vi "BGAndSrewImage.vi"(8 "error in (no error)":errorcluster, 9 "BG Image":T1, 10 "Image":T1, 11 "S arrays.S 0":i32[][](array[numeric])) -> (0 "error out":errorcluster, 1 "empty image":bool, 3 "Image Out":T1, 4 "time 2":u32)   [LabVIEW 2011]
uses:
  IMAQ Image.ctl
  NI_Vision_Development_Module.lvlib
panel:
  out "time:filter":u32
  out "time:screw":u32
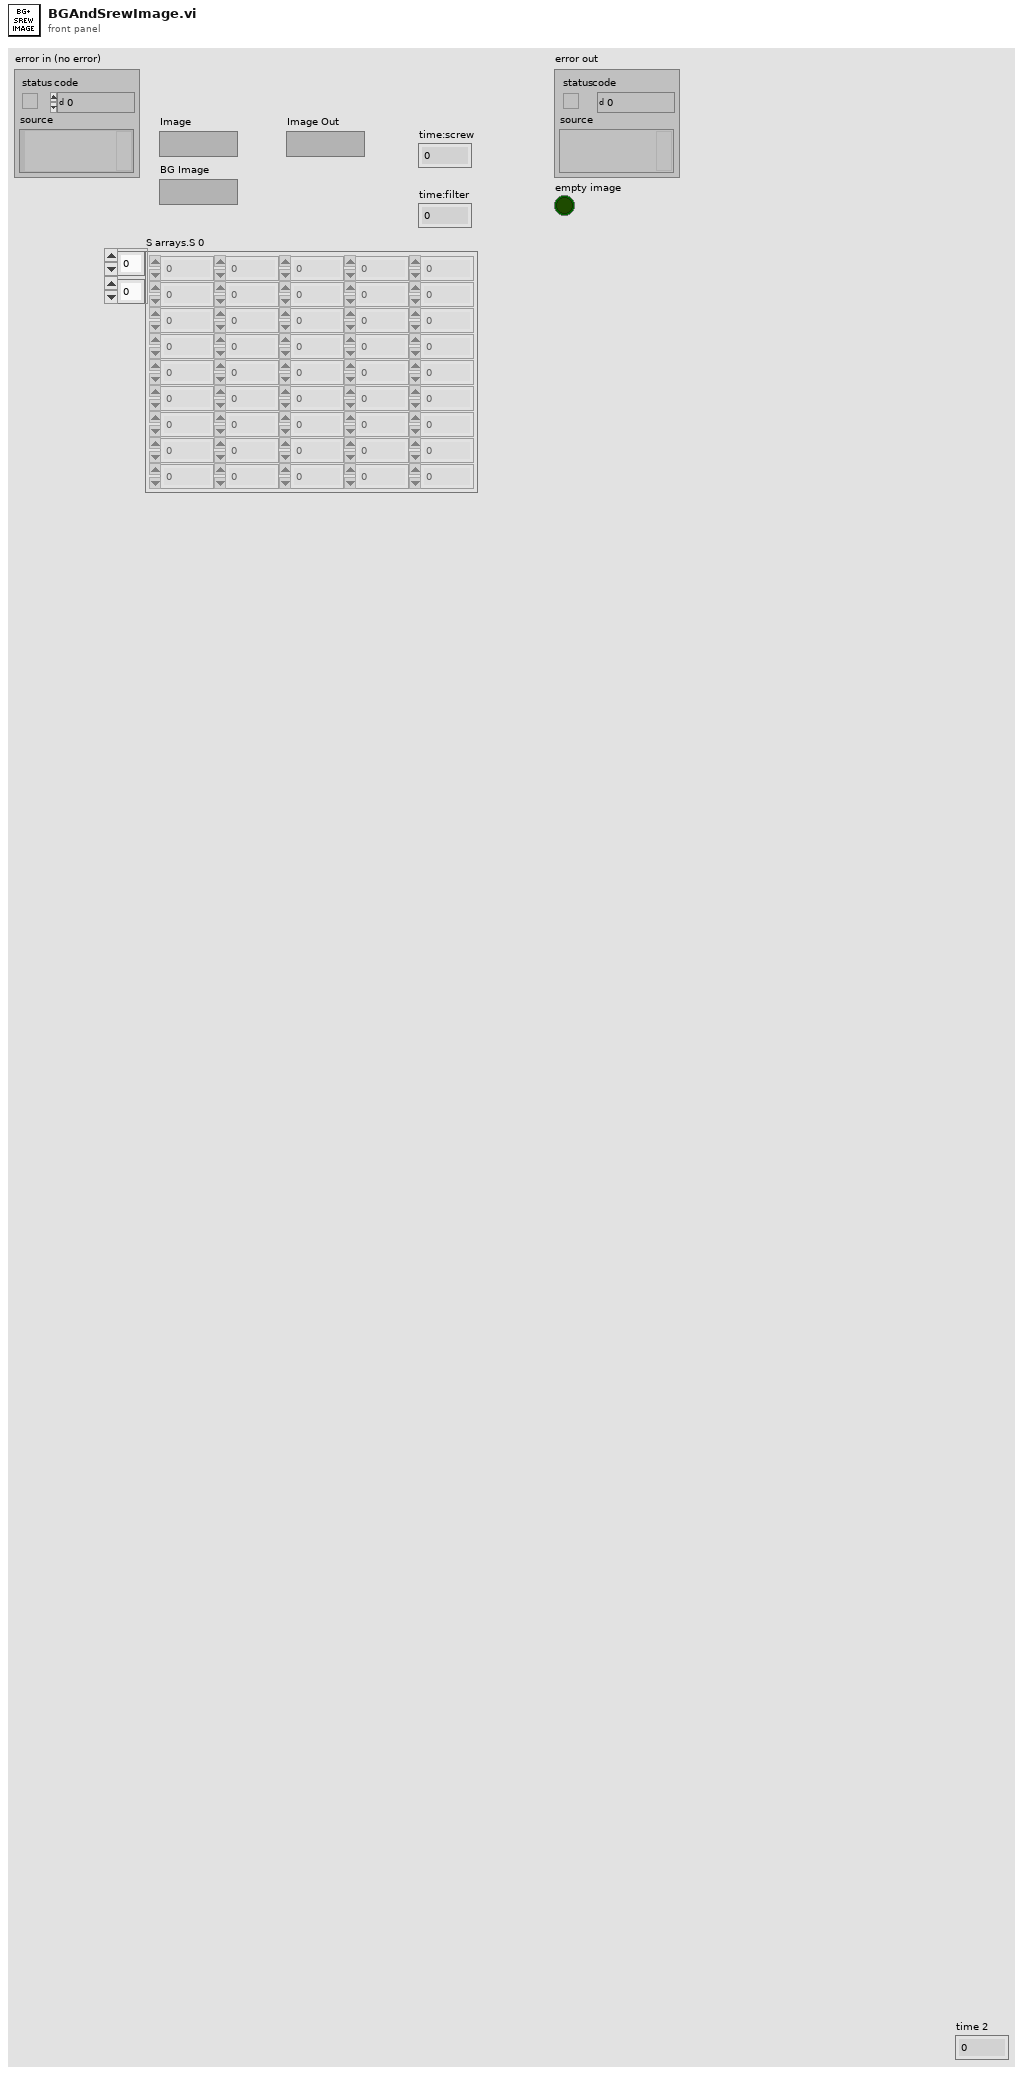
[diagram p1: front panel]
types:
  T1 = typedef "IMAQ Image.ctl" = refnum<image>
  T2 = cluster{"X Size":i32, "Y Size":i32, "Order #":i32}
  T3 = cluster{"X Size":i32, "Y Size":i32, "% Tolerance":i32}
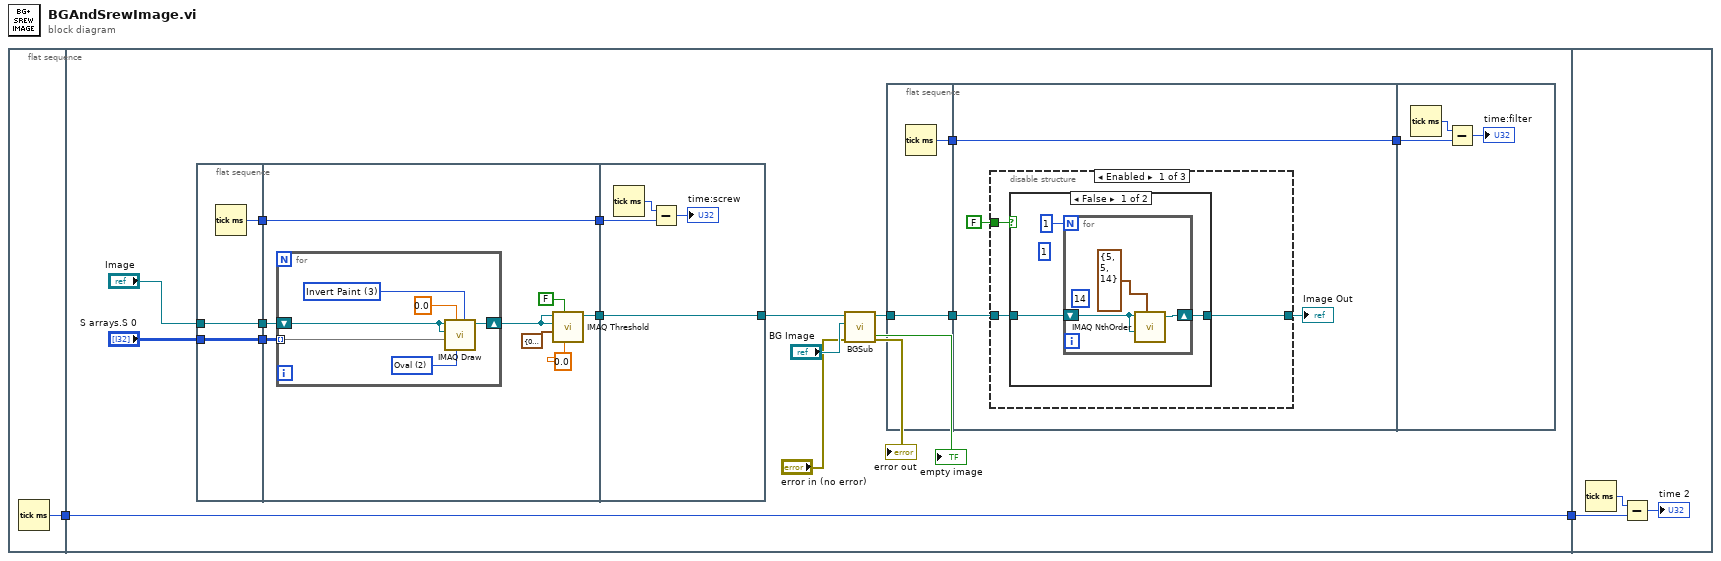
[diagram p0: block diagram]
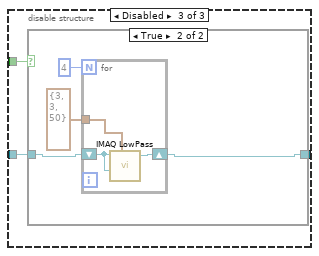
[diagram p4: hidden frame]
diagram:
  n1 = flat-sequence {
    tunnel: [w3] -> w1
    tunnel: [w19] -> w2
    tunnel: w1 -> [w19]
    tunnel: w2 -> [w73]
    frame #0 {
      n2 = Tick Count (ms)() -> (millisecond timer value=w3:u32)
    }
    frame #1 {
      n3 = flat-sequence {
        tunnel: "Image" -> [w53]
        tunnel: "S arrays.S 0" -> [w54]
        tunnel: [w54] -> w17
        tunnel: [w53] -> w16
        tunnel: [w52] -> w15
        tunnel: [w56] -> w18
        tunnel: w17 -> [w62]
        tunnel: w16 -> [w61]
        tunnel: w15 -> [w55]
        tunnel: [w55] -> w14
        tunnel: [w72] -> w10
        tunnel: w18 -> [w72]
        tunnel: w14 -> [w69]
        frame #0 {
          n4 = Tick Count (ms)() -> (millisecond timer value=w52:u32)
        }
        frame #1 {
          n5 = for {
            shift-right: [w67] -> w57
            shift-left: w61 -> [w68]
            tunnel: w62 -> [w64] mode=indexing
            w66 = u16 2 items=["Line", "Rectangle", "Oval"] ("Shape to draw")
            w65 = u16 3 items=["Frame", "Paint", "Invert Frame", "Invert Paint"] ("Draw Mode")
            n6 = call "IMAQ Draw"("Draw Mode"=w65, "Shape to draw"=w66, "Pixel Color"=sgl 0.0, "Coordinates"=w64, "Image Dst"=w68, "Image Src"=w68) -> ("Image Dst Out"=w67:T1)  [unwired: 4 in, 1 out]
          }
          n7 = call "IMAQ Threshold"("Replace Value"=sgl 0.0, "Keep/Replace Value (Replace)"=FALSE, "Range"=cluster{"Lower value":sgl, "Upper value":sgl} {"Lower value"=0.0, "Upper value"=999999.0}, "Image Dst"=w57, "Image Src"=w57) -> ("Image Dst Out"=w56:T1)  [unwired: 5 in, 1 out]
        }
        frame #2 {
          n8 = Tick Count (ms)() -> (millisecond timer value=w70:u32)
          n9 = Subtract(x=w70, y=w69) -> (x-y=→"time:screw":u32)
        }
      }
      n10 = call "BGSub.vi"("error in (no error)"="error in (no error)", "BG IN"="BG Image", "raw Image In"=w10) -> ("error out"=→"error out":errorcluster, "Refnum out"=w9:T1, "empty image"=→"empty image":bool)  [unwired: 6 in]
      n11 = flat-sequence {
        tunnel: w9 -> [w22]
        tunnel: [w22] -> w13
        tunnel: [w21] -> w11
        tunnel: w13 -> [w24]
        tunnel: [w26] -> w12
        tunnel: w11 -> [w26]
        tunnel: w12 -> [w49]
        frame #0 {
          n12 = Tick Count (ms)() -> (millisecond timer value=w21:u32)
        }
        frame #1 {
          n13 = disable-structure shown="Enabled" {
            disable-tunnel: [w28 w37 w39] -> w25
            disable-tunnel: w24 -> [w29 w37 w40]
            disable-tunnel: FALSE ("empty array") -> [w27 _ w38]
            frame Enabled {
              n14 = case shown="False" w27 {
                tunnel: w29 -> [w32 w36]
                tunnel: [w31 w36] -> w28
                frame False {
                  (unwired) 1
                  n15 = for {
                    N: 1 -> [_]
                    shift-right: [w33] -> w31
                    shift-left: w32 -> [w35]
                    (unwired) 14 ("Order #")
                    n16 = call "IMAQ NthOrder"("Image Src"=w35, "Size & Order #"=T2 {"X Size"=5, "Y Size"=5, "Order #"=14}, "Image Dst"=w35) -> ("Image Dst Out"=w33:T1)  [unwired: 4 in, 1 out]
                  }
                }
                frame True {
                }
              }
            }
            frame Disabled {
            }
            frame Disabled {
              n17 = case shown="True" w38 {
                tunnel: w40 -> [w41 w42]
                tunnel: [w41 w43] -> w39
                frame False {
                }
                frame True {
                  n18 = for {
                    N: 4 -> [_]
                    tunnel: T3 {"X Size"=3, "Y Size"=3, "% Tolerance"=50} ("Size & Tolerance") -> [w47]
                    shift-right: [w46] -> w43
                    shift-left: w42 -> [w48]
                    n19 = call "IMAQ LowPass"("Image Src"=w48, "Size & Tolerance"=w47, "Image Dst"=w48) -> ("Image Dst Out"=w46:T1)  [unwired: 4 in, 1 out]
                  }
                }
              }
            }
          }
          "Image Out" <- w25
        }
        frame #2 {
          n20 = Tick Count (ms)() -> (millisecond timer value=w51:u32)
          n21 = Subtract(x=w51, y=w49) -> (x-y=→"time:filter":u32)
        }
      }
    }
    frame #2 {
      n22 = Tick Count (ms)() -> (millisecond timer value=w74:u32)
      n23 = Subtract(x=w74, y=w73) -> (x-y=→"time 2":u32)
    }
  }
